vi "Record and playback example for pco.cameras with CamRam.vi"() -> ()   [LabVIEW 2012]
doc: "A short program to demonstrate the fundamentals of control and image acquision with the pco.camera series. The program records a sequence of images, with \"live\" updating, until the \"StopRecording\" button is pressed. A subset of recorded images is then read out from the camera RAM. Warning: Limit the number of images read back tfrom the camera RAM to a reasonable number. Images are stored as a three-dimensional array, which can very large. Use ctrl-H for more help on the individual controls and indicators.\n\nCopyright 2004, the Cooke Corporation."
panel:
  out "bClose":bool
  in  "Quit":bool
  in  "ImageNr":i32
  in  "Image":i32
  out "BufNr1":i16
  out "BufNr0":i16
  in  "bUseBuffer1":bool
  in  "bUseBuffer0":bool
  in  "ROIX1":u16=1 min=1
  in  "ROIY1":u16=1 min=1
  in  "ROIY0":u16=1 min=1
  in  "ROIX0":u16=1 min=1
  out "Bits/pixel":u16
  in  "Readout":bool
  in  "Record":bool
  in  "Stop":u32=10 min=1
  in  "Start":u32=1 min=1
  in  "DelayTimeBase":u16(ring)=2 items=["nanoseconds", "microseconds", "milliseconds"]
  in  "ExposureTimeBase":u16(ring)=2 items=["nanoseconds", "microseconds", "milliseconds"]
  in  "Exposure":u32=10
  in  "Delay":u32
  out "Reading":bool
  in  "StorageMode":bool
  out "ImageCount":u32
  in  "Rate":i32
  out "Image":u16[][](graph)
  in  "TriggerMode":u16(ring) items=["Auto", "Software", "External sequence start ", "External exposure control"]
  # "A short program to demonstrate the fundamentals of control and image acquision with the pco.camera series. The program records a sequence of images, with \"live\" updating, until the \"StopRecording\" button is pressed. A subset of recorded images is then read out from the camera RAM. WARNING: Limit the number of images read back tfrom the camera RAM to a reasonable number. Images are stored as a three-dimensional array, which can very large.  Use ctrl-H for more help on the individual controls and indicators."
  # "pco.labview"
  # "1) Setup camera:"
  # "FIFO"
  # "Recorder"
  # "2) Record  images:"
  # "3) Read out images:"
  # "4) Display image:"
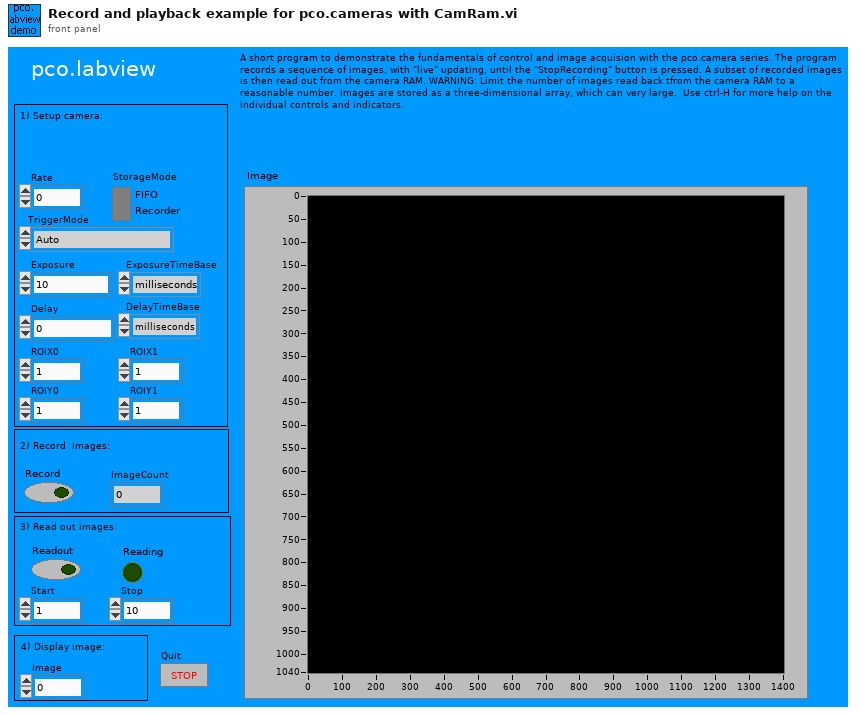
[diagram p1: front panel]
types:
  T1 = cluster{"Size":u16, "CamType":u16, "CamSubType":u16, "SerialNumber":u32, "HWVersion":u32, "FWVersion":u32, "InterfaceType":u16, "HardwareVersion":cluster{"BoardNum":u16, "HWVersions":cluster{"BoardName":string, "BatchNumber":u16, "MinorRevision":u8, "MajorRevision":u8, "Variant":u16}[]}, "FirmwareVersion":cluster{"DeviceNum":u16, "FWVersions":cluster{"DeviceName":string, "MinorRevision":u8, "MajorRevision":u8, "Variant":u16}[]}}
  T2 = cluster{"Size":u16, "SensorTypeDESC":u16, "SensorSubtypeDESC":u16, "MaxHorizontalResStdDESC":u16, "MaxVerticalResStdDESC":u16, "MaxHorizontalResExtDESC":u16, "MaxVerticalResExtDESC":u16, "DynResDESC":u16, "MaxBinHorzDESC":u16, "BinHorzStepDESC":bool, "MaxBinVertDESC":u16, "BinVertStepDESC":bool, "ROIHorzStepDESC":u16, "ROIVertStepDESC":u16, "NumADCDESC":u16, "IRDESC":bool, "MinDelayDESC":u32, "MaxDelayDESC":u32, "MinDelayStepDESC":u32, "MinExpoDESC":u32, "MaxExpoDESC":u32, "MinExpoStepDESC":u32, "MinDelayIRDESC":u32, "MaxDelayIRDESC":u32, "MinExpoIRDESC":u32, "MaxExpoIRDESC":u32, "TimeTableDESC":bool, "DoubleImageDESC":bool, "MinCoolSetDESC":i16, "MaxCoolSetDESC":i16, "MDefaultCoolSetDESC":i16, "PowerDownModeDESC":bool, "OffsetRegDESC":bool, "ColorPattern":cluster{"UpperLeftColor":u8, "UpperRightColor":u8, "LowerLeftColor":u8, "LowerRightColor":u8}, "PatternTypeDESC":bool, "PixelRates":u32[], "CoversionFactors":u16[], "Reserved":u32[], "NoiseFilterCapable":bool, "HotPixelCapable":bool, "HotPixelWithNoiseFilter":bool, "ASCIITimeCapable":bool, "Extended Description":bool, "Get Extended":bool, "Reserved Flag 1":bool, "Reserved Flag 2":bool}
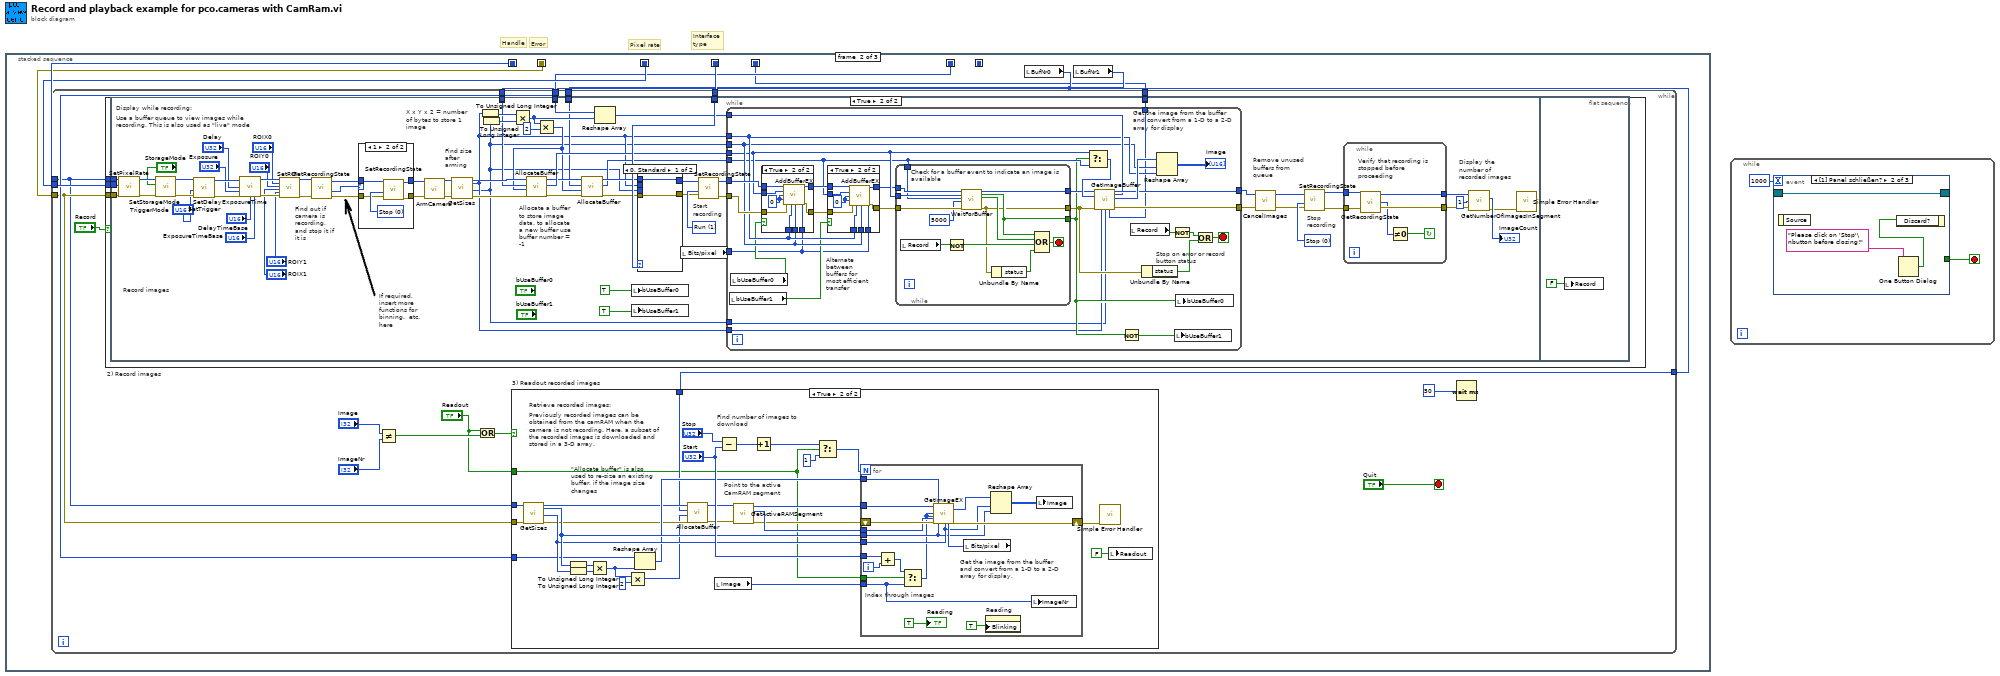
[diagram p0: block diagram]
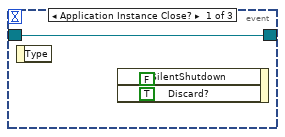
[diagram p2: hidden frame]
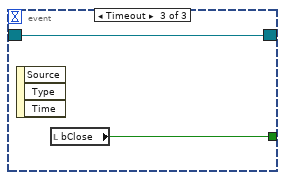
[diagram p3: hidden frame]
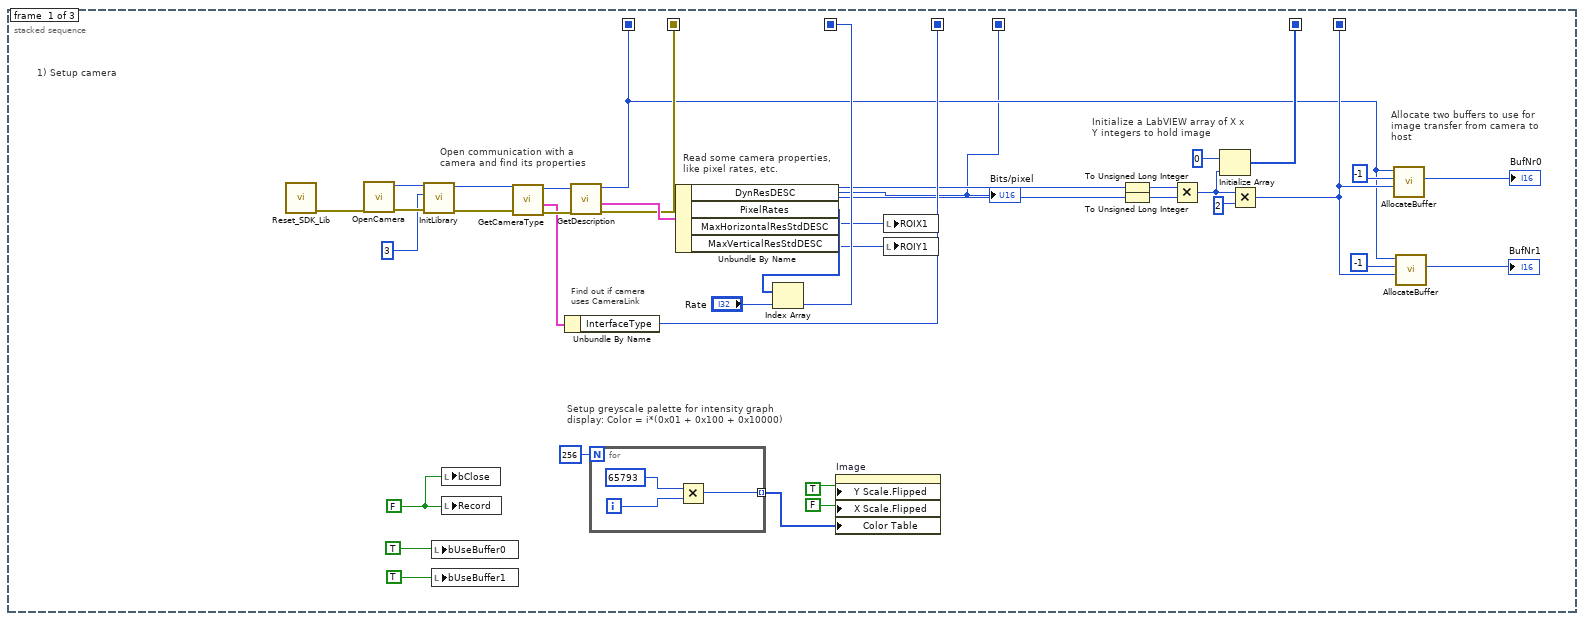
[diagram p4: hidden frame]
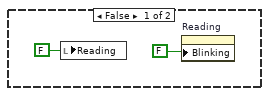
[diagram p5: hidden frame]
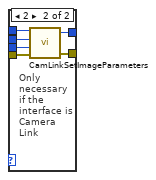
[diagram p9: hidden frame]
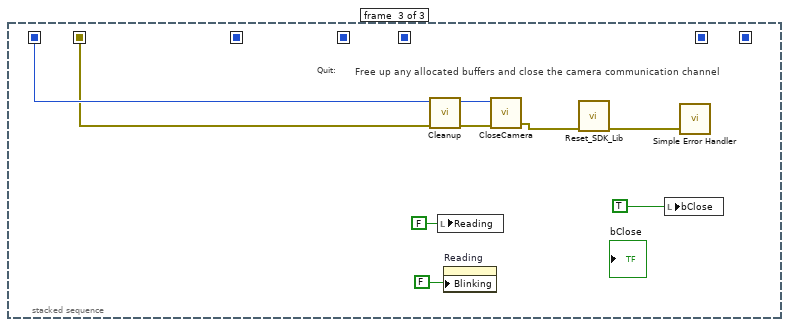
[diagram p11: hidden frame]
diagram:
  # "Interface type"
  # "Error"
  # "Handle"
  # "Pixel rate"
  n1 = stacked-sequence {
    seq-local: [w31 _ _] -> [_ w44 _]
    seq-local: [w15 _ _] -> [_ _ _]
    seq-local: [w23 _ _] -> [_ w46 _]
    seq-local: [w14 _ _] -> [_ w48 w285]
    seq-local: [w22 _ _] -> [_ w47 w284]
    seq-local: [w21 _ _] -> [_ w45 _]
    seq-local: [w1 _ _] -> [_ w41 _]
    frame #0 {
      w8 = FALSE ("stop")
      # "Read some camera properties, like pixel rates, etc."
      # "Allocate two buffers to use for image transfer from camera to host"
      # "1) Setup camera"
      # "Find out if camera uses CameraLink"
      # "Setup greyscale palette for intensity graph display: Color = i*(0x01 + 0x100 + 0x10000)"
      # "Initialize a LabVIEW array of X x Y integers to hold image"
      # "Open communication with a camera and find its properties"
      n2 = call "Reset_SDK_Lib.vi"() -> ("ErrorOut"=w4:errorcluster)  [unwired: 11 in]
      n3 = call "OpenCamera.vi"("ErrorIn"=w4) -> ("ErrorOut"=w6:errorcluster, "Handle out"=w7:u64)  [unwired: 3 in, 2 out]
      n4 = call "InitLibrary.vi"("error in (no error)"=w6, "InterfaceType"=u32 3, "ph"=w7) -> ("error out"=w2:errorcluster, "hout"=w3:u64)  [unwired: 7 in]
      n5 = local write "bUseBuffer0"(TRUE) -> ()
      n6 = local write "bUseBuffer1"(TRUE) -> ()
      n7 = local write "bClose"(w8) -> ()
      n8 = local write "Record"(w8) -> ()
      n9 = call "GetCameraType.vi"("ph"=w3, "error in (no error)"=w2) -> ("hout"=w27:u64, "CameraType"=w25:T1, "error out"=w26:errorcluster)  [unwired: 1 in, 1 out]
      n10 = Unbundle By Name(w25) -> ("InterfaceType"=w21:u16)
      n11 = call "GetDescription.vi"("ErrorIn"=w26, "ph"=w27) -> ("ErrorOut"=w22:errorcluster, "Description"=w30:T2, "hout"=w14:u64)  [unwired: 2 in, 1 out]
      n12 = for {
        N: 256 -> [_]
        tunnel: [w38] -> w34 mode=indexing
        i -> [w39]
        n13 = Multiply(x=65793, y=w39) -> (x*y=w38:i32)
      }
      n14 = Unbundle By Name(w30) -> ("DynResDESC"=w1:u16, "PixelRates"=w24:u32[], "MaxHorizontalResStdDESC"=w20:u16, "MaxVerticalResStdDESC"=w19:u16)
      "Bits/pixel" <- w1
      n15 = Index Array(array=w24, index="Rate") -> (element=w23:u32)
      n16 = property on="Image" class="IntGraph (strikt)"("Y Scale.Flipped"=TRUE, "X Scale.Flipped"=FALSE, "Color Table"=w34) -> ()  [unwired: 2 in, 2 out]
      n17 = local write "ROIX1"(w20) -> ()
      n18 = local write "ROIY1"(w19) -> ()
      n19 = To Unsigned Long Integer(number=w20) -> (unsigned 32bit integer=w17:u32)
      n20 = To Unsigned Long Integer(number=w19) -> (unsigned 32bit integer=w16:u32)
      n21 = Multiply(x=w17, y=w16) -> (x*y=w32:u32)
      n22 = Initialize Array(u16 0 ("Element Data"), w32) -> (w31:u16[])
      n23 = Multiply(x=w32, y=u32 2) -> (x*y=w15:u32)
      n24 = call "AllocateBuffer.vi"("Size"=w15, "BufNr"=i16 -1, "ph"=w14) -> ("BufNrOut"=→"BufNr0":i16)  [unwired: 3 in, 5 out]
      n25 = call "AllocateBuffer.vi"("Size"=w15, "BufNr"=-1, "ph"=w14) -> ("BufNrOut"=→"BufNr1":i16)  [unwired: 3 in, 5 out]
    }
    frame #1 {
      n26 = local read "BufNr0"() -> (w43:i16)
      n27 = local read "BufNr1"() -> (w42:i16)
      n28 = while {
        tunnel: w43 -> [w58]
        tunnel: w43 -> [w59]
        tunnel: w44 -> [w61]
        tunnel: w45 -> [w62]
        tunnel: w46 -> [w63]
        tunnel: w47 -> [w60]
        tunnel: w48 -> [w56]
        tunnel: w42 -> [w57]
        tunnel: w41 -> [w49]
        stop <- "Quit" stop-if-true
        n29 = case "2) Record images" shown="True" "Record" {
          tunnel: w56 -> [_ w122]
          tunnel: w60 -> [_ w121]
          tunnel: w63 -> [_ w120]
          tunnel: w62 -> [_ w119]
          tunnel: w61 -> [_ w118]
          tunnel: w59 -> [_ w117]
          tunnel: w57 -> [_ w116]
          tunnel: w49 -> [_ w115]
          frame False {
          }
          frame True {
            n30 = flat-sequence {
              tunnel: w122 -> [w166]
              tunnel: w121 -> [w165]
              tunnel: w120 -> [w163]
              tunnel: w119 -> [w162]
              tunnel: w118 -> [w160]
              tunnel: w117 -> [w145]
              tunnel: w116 -> [w139]
              tunnel: w115 -> [w123]
              frame #0 {
                w190 = u16 1 items=["Stop", "Run"] ("RecordingState")
                w193 = u16 0 items=["Stop", "Run"] ("RecordingState")
                # "Remove unused buffers from queue"
                # "Display the number of recorded images"
                # "Record images"
                # "Start recording"
                # "Allocate a buffer to store image data. to allocate a new buffer use buffer number = -1"
                # "Find size after arming"
                # "Find out if camera is recording, and stop it if it is"
                # "If required, insert more functions for binning.  etc. here"
                # "X x Y x 2 = number of bytes to store 1 image"
                # "Stop recording"
                # "Use a buffer queue to view images while recording. This is also used as \"live\" mode"
                # "Display while recording:"
                n31 = call "SetPixelRate.vi"("error in (no error)"=w165, "PixelRate"=w163, "ph"=w166) -> ("error out"=w188:errorcluster, "hout"=w189:u64)  [unwired: 2 in, 1 out]
                n32 = call "SetStorageMode.vi"("error in (no error)"=w188, "StorageMode"="StorageMode", "ph"=w189) -> ("error out"=w180:errorcluster, "hout"=w181:u64)  [unwired: 2 in, 1 out]
                n33 = call "SetTrigger.vi"("error in (no error)"=w180, "TriggerMode"="TriggerMode", "ph"=w181) -> ("error out"=w173:errorcluster, "hout"=w174:u64)  [unwired: 2 in, 1 out]
                n34 = call "SetDelayExposureTime.vi"("ph"=w174, "Delay"="Delay", "Exposure"="Exposure", "error in (no error)"=w173, "DelayTimeBase"="DelayTimeBase", "ExposureTimeBase"="ExposureTimeBase") -> ("hout"=w153:u64, "error out"=w151:errorcluster)  [unwired: 7 in, 1 out]
                n35 = call "SetROI.vi"("ph"=w153, "ROIX0"="ROIX0", "ROIY0"="ROIY0", "ROIX1"="ROIX1", "ROIY1"="ROIY1", "error in (no error)"=w151) -> ("hout"=w152:u64, "error out"=w150:errorcluster)  [unwired: 12 in]
                n36 = call "GetRecordingState.vi"("ErrorIn"=w150, "ph"=w152) -> ("ErrorOut"=w184:errorcluster, "RecordingState"=w186:u16, "hout"=w185:u64)  [unwired: 2 in, 1 out]
                n37 = case shown="1" w186 {
                  tunnel: w185 -> [w274 w278]
                  tunnel: w184 -> [w273 w277]
                  tunnel: [w274 w276] -> w183
                  tunnel: [w273 w275] -> w182
                  frame 0, Default {
                  }
                  frame 1 {
                    w279 = u16 0 items=["Stop", "Run"] ("RecordingState")
                    n38 = call "SetRecordingState.vi"("ErrorIn"=w277, "RecordingState"=w279, "ph"=w278) -> ("ErrorOut"=w275:errorcluster, "hout"=w276:u64)  [unwired: 2 in, 1 out]
                  }
                }
                n39 = call "ArmCamera.vi"("error in (no error)"=w182, "ph"=w183) -> ("error out"=w178:errorcluster, "hout"=w179:u64)  [unwired: 1 in, 1 out]
                n40 = call "GetSizes.vi"("ph"=w179, "ErrorIn"=w178) -> ("hout"=w175:u64, "XResAct"=w125:u16, "YResAct"=w124:u16, "ErrorOut"=w177:errorcluster)  [unwired: 11 in, 3 out]
                n41 = To Unsigned Long Integer(number=w125) -> (unsigned 32bit integer=w154:u32)
                n42 = To Unsigned Long Integer(number=w124) -> (unsigned 32bit integer=w155:u32)
                n43 = Multiply(x=w154, y=w155) -> (x*y=w156:u32)
                n44 = Multiply(x=w156, y=u32 2) -> (x*y=w140:u32)
                n45 = call "AllocateBuffer.vi"("error in (no error)"=w177, "Size"=w140, "BufNr"=w145, "ph"=w175) -> ("error out"=w144:errorcluster, "BufNrOut"=w157:i16, "hout"=w142:u64)  [unwired: 2 in, 3 out]
                n46 = call "AllocateBuffer.vi"("error in (no error)"=w144, "Size"=w140, "BufNr"=w139, "ph"=w142) -> ("error out"=w143:errorcluster, "BufNrOut"=w138:i16, "hout"=w141:u64)  [unwired: 2 in, 3 out]
                n47 = Reshape Array(w160, w156) -> (w159:u16[])
                n48 = local write "bUseBuffer0"(TRUE) -> ()
                n49 = local write "bUseBuffer1"(TRUE) -> ()
                n50 = case shown="0, Standard" w162 {
                  tunnel: w143 -> [w265 w272]
                  tunnel: [w265 w271] -> w168
                  tunnel: w141 -> [w266 w270]
                  tunnel: [w266 w269] -> w167
                  tunnel: w124 -> [_ w268]
                  tunnel: w125 -> [_ w267]
                  frame 0, Default {
                  }
                  frame 2 {
                    # "Only necessary if the interface is Camera Link"
                    n51 = call "CamLinkSetImageParameters.vi"("error in (no error)"=w272, "YRes"=w268, "XRes"=w267, "ph"=w270) -> ("error out"=w271:errorcluster, "hout"=w269:u64)  [unwired: 1 out]
                  }
                }
                n52 = local read "Bits/pixel"() -> (w131:u16)
                n53 = call "SetRecordingState.vi"("ErrorIn"=w168, "RecordingState"=w190, "ph"=w167) -> ("ErrorOut"=w164:errorcluster, "hout"=w161:u64)  [unwired: 2 in, 1 out]
                n54 = while {
                  tunnel: w157 -> [w206]
                  tunnel: w159 -> [w219]
                  tunnel: w161 -> [w218]
                  tunnel: w124 -> [w213]
                  tunnel: w125 -> [w214]
                  tunnel: w164 -> [w216]
                  tunnel: [w221] -> w130
                  tunnel: [w222] -> w129
                  tunnel: w138 -> [w205]
                  tunnel: w131 -> [w209]
                  tunnel: w125 -> [w196]
                  tunnel: w124 -> [w195]
                  tunnel: w123 -> [w194]
                  stop <- w197 stop-if-true
                  # "Alternate between buffers for most efficient transfer"
                  # "Stop on error or record button status"
                  # "Get the image from the buffer and convert from a 1-D to a 2-D array for display"
                  n55 = local read "bUseBuffer1"() -> (w211:bool)
                  n56 = local read "bUseBuffer0"() -> (w212:bool)
                  n57 = case shown="True" w212 {
                    tunnel: [w225 w234] -> w215
                    tunnel: [w224 w233] -> w217
                    tunnel: w206 -> [_ w232]
                    tunnel: w218 -> [w224 w231]
                    tunnel: w209 -> [_ w229]
                    tunnel: w214 -> [_ w228]
                    tunnel: w213 -> [_ w227]
                    tunnel: w216 -> [w225 w226]
                    frame False {
                    }
                    frame True {
                      w230 = 0
                      n58 = call "AddBufferEX.vi"("ph"=w231, "BuffNr"=w232, "1stImage"=w230, "LastImage"=w230, "error in (no error)"=w226, "XRes"=w228, "YRes"=w227, "BitPerPixel"=w229) -> ("hout"=w233:u64, "error out"=w234:errorcluster)  [unwired: 5 in, 1 out]
                    }
                  }
                  n59 = case shown="True" w211 {
                    tunnel: [w235 w245] -> w203
                    tunnel: [w236 w244] -> w204
                    tunnel: w205 -> [_ w243]
                    tunnel: w217 -> [w236 w242]
                    tunnel: w209 -> [_ w240]
                    tunnel: w214 -> [_ w239]
                    tunnel: w213 -> [_ w238]
                    tunnel: w215 -> [w235 w237]
                    frame False {
                    }
                    frame True {
                      w241 = 0
                      n60 = call "AddBufferEX.vi"("ph"=w242, "BuffNr"=w243, "1stImage"=w241, "LastImage"=w241, "error in (no error)"=w237, "XRes"=w239, "YRes"=w238, "BitPerPixel"=w240) -> ("hout"=w244:u64, "error out"=w245:errorcluster)  [unwired: 5 in, 1 out]
                    }
                  }
                  n61 = while {
                    tunnel: w206 -> [w253]
                    tunnel: w205 -> [w252]
                    tunnel: w204 -> [w255]
                    tunnel: w203 -> [w254]
                    tunnel: [w251] -> w202
                    tunnel: [w247] -> w200
                    tunnel: [w250] -> w201
                    stop <- w256 stop-if-true
                    # "Check for a buffer event to indicate an image is available"
                    n62 = local read "Record"() -> (w258:bool)
                    n63 = Not(x=w258) -> (.not. x?=w257:bool)
                    n64 = call "WaitForBuffer.vi"("ph"=w255, "sBufNr"=w253, "sBufNr 2"=w252, "timeout"=5000, "error in (no error)"=w254) -> ("hout"=w251:u64, "Buffer_Ready"=w250:bool, "Buffer_Ready 2"=w249:bool, "error out"=w247:errorcluster)  [unwired: 10 in, 1 out]
                    n65 = Unbundle By Name(w247) -> ("status"=w246:bool)
                    n66 = Compound Arithmetic op=OR(w250, w249, w257, w246) -> (w256:bool)
                  }
                  n67 = Select(t=w206, s=w201, f=w205) -> (s? t:f=w210:i16)
                  n68 = call "GetImageBuffer.vi"("ph"=w202, "BuffIn"=w219, "BuffNr"=w210, "error in (no error)"=w200, "xRes"=w196, "yRes"=w195, "Bitresolution"=w194) -> ("hout"=w221:u64, "BuffOut"=w223:u16[], "error out"=w222:errorcluster)  [unwired: 5 in, 1 out]
                  n69 = Not(x=w201) -> (.not. x?=w208:bool)
                  n70 = local read "Record"() -> (w220:bool)
                  n71 = Unbundle By Name(w200) -> ("status"=w198:bool)
                  n72 = Reshape Array(w223, w213, w214) -> (→"Image":u16[][])
                  n73 = Not(x=w220) -> (.not. x?=w199:bool)
                  n74 = local write "bUseBuffer1"(w208) -> ()
                  n75 = local write "bUseBuffer0"(w201) -> ()
                  n76 = Or(x=w199, y=w198) -> (x .or. y?=w197:bool)
                }
                n77 = call "CancelImages.vi"("error in (no error)"=w129, "ph"=w130) -> ("error out"=w135:errorcluster, "hout"=w134:u64)  [unwired: 1 in, 1 out]
                n78 = call "SetRecordingState.vi"("ErrorIn"=w135, "RecordingState"=w193, "ph"=w134) -> ("ErrorOut"=w191:errorcluster, "hout"=w192:u64)  [unwired: 2 in, 1 out]
                n79 = while {
                  tunnel: [w262] -> w128
                  tunnel: w191 -> [w263]
                  tunnel: w192 -> [w264]
                  tunnel: [w259] -> w127
                  stop <- w260 continue-if-true
                  # "Verify that recording is stopped before proceeding"
                  n80 = call "GetRecordingState.vi"("ErrorIn"=w263, "ph"=w264) -> ("ErrorOut"=w262:errorcluster, "RecordingState"=w261:u16, "hout"=w259:u64)  [unwired: 2 in, 1 out]
                  n81 = Not Equal To 0?(x=w261) -> (x != 0?=w260:bool)
                }
                n82 = call "GetNumberOfImagesInSegment.vi"("ph"=w127, "Segment"=u16 1, "error in (no error)"=w128) -> ("ValidImageCnt"=→"ImageCount":u32, "error out"=w126:errorcluster)  [unwired: 3 out]
                n83 = call <vilib>:"Simple Error Handler.vi"("error in (no error)"=w126) -> ()  [unwired: 4 in, 5 out]
              }
              frame #1 {
                n84 = local write "Record"(FALSE ("Record")) -> ()
              }
            }
          }
        }
        n85 = Not Equal?(x="Image", y="ImageNr") -> (x != y?=w53:bool)
        n86 = Or(x="Readout", y=w53) -> (x .or. y?=w52:bool)
        n87 = case "3) Readout recorded images" shown="True" w52 {
          tunnel: w61 -> [_ w89]
          tunnel: w56 -> [_ w81]
          tunnel: w60 -> [_ w80]
          tunnel: w58 -> [_ w74]
          tunnel: "Readout" -> [_ w68]
          frame False {
            n88 = local write "Reading"(FALSE ("Reading")) -> ()
            n89 = property on="Reading" class="Bool. (strikt)"("Blinking"=FALSE) -> ()  [unwired: 2 in, 2 out]
          }
          frame True {
            # "Point to the active CamRAM segment"
            # "\"Allocate buffer\" is also used to re-size an existing buffer, if the image size changes"
            # "Find number of images to download"
            # "Previously recorded images can be obtained from the camRAM when the camera is not recording. Here, a subset of the recorded images is downloaded and stored in a 3-D array."
            # "Retrieve recorded images:"
            n90 = call "GetSizes.vi"("ph"=w81, "ErrorIn"=w80) -> ("hout"=w87:u64, "XResAct"=w91:u16, "YResAct"=w90:u16, "ErrorOut"=w85:errorcluster)  [unwired: 11 in, 3 out]
            n91 = To Unsigned Long Integer(number=w91) -> (unsigned 32bit integer=w77:u32)
            n92 = To Unsigned Long Integer(number=w90) -> (unsigned 32bit integer=w78:u32)
            n93 = Multiply(x=w77, y=w78) -> (x*y=w79:u32)
            n94 = Multiply(x=w79, y=u32 2) -> (x*y=w76:u32)
            n95 = Reshape Array(w89, w79) -> (w88:u16[])
            n96 = call "AllocateBuffer.vi"("error in (no error)"=w85, "Size"=w76, "BufNr"=w74, "ph"=w87) -> ("error out"=w84:errorcluster, "hout"=w86:u64)  [unwired: 2 in, 4 out]
            n97 = local read "Image"() -> (w72:i32)
            n98 = Subtract(x="Stop", y="Start") -> (x-y=w95:u32)
            n99 = call "GetActiveRAMSegment.vi"("error in (no error)"=w84, "ph"=w86) -> ("error out"=w82:errorcluster, "ActSeg"=w92:u16, "hout"=w83:u64)  [unwired: 2 in, 1 out]
            n100 = Increment(x=w95) -> (x+1=w71:u32)
            n101 = Select(t=w71, s=w68, f=1) -> (s? t:f=w70:u32)
            n102 = for {
              N: w70 -> [_]
              tunnel: w83 -> [w114]
              shift-right: [w111] -> w73
              shift-left: w82 -> [w110]
              tunnel: "Start" -> [w107]
              tunnel: w92 -> [w105]
              tunnel: w91 -> [w101]
              tunnel: w90 -> [w102]
              tunnel: w88 -> [w103]
              tunnel: w72 -> [w97]
              tunnel: w68 -> [w99]
              i -> [w106]
              # "Get the image from the buffer and convert from a 1-D to a 2-D array for display."
              # "Index through images"
              n103 = Add(x=w107, y=w106) -> (x+y=w98:u32)
              n104 = Select(t=w98, s=w99, f=w97) -> (s? t:f=w100:u32)
              n105 = local read "Bits/pixel"() -> (w104:u16)
              n106 = call "GetImageEX.vi"("ph"=w114, "1stImage"=w100, "lastImage"=w100, "segment"=w105, "error in (no error)"=w110, "BuffIn"=w103, "xRes"=w101, "yRes"=w102, "BitPerPixel"=w104) -> ("BuffOut"=w113:u16[], "error out"=w111:errorcluster)  [unwired: 7 in, 2 out]
              n107 = property on="Reading" class="Bool. (strikt)"("Blinking"=TRUE) -> ()  [unwired: 2 in, 2 out]
              n108 = Reshape Array(w113, w102, w101) -> (w112:u16[][])
              n109 = local write "ImageNr"(w97) -> ()
              n110 = local write "Image"(w112) -> ()
              "Reading" <- TRUE ("Reading")
            }
            n111 = call <vilib>:"Simple Error Handler.vi"("error in (no error)"=w73) -> ()  [unwired: 4 in, 5 out]
            n112 = local write "Readout"(FALSE ("Readout")) -> ()
          }
        }
        n113 = Wait (ms)(milliseconds to wait=u32 50) -> ()  [unwired: 1 out]
      }
    }
    frame #2 {
      # "Free up any allocated buffers and close the camera communication channel"
      # "Quit:"
      n114 = call "Cleanup.vi"("error in (no error)"=w284, "ph"=w285) -> ("error out"=w283:errorcluster, "hout"=w282:u64)  [unwired: 8 in]
      n115 = local write "Reading"(FALSE ("Reading")) -> ()
      n116 = property on="Reading" class="Bool. (strikt)"("Blinking"=FALSE) -> ()  [unwired: 2 in, 2 out]
      n117 = call "CloseCamera.vi"("ErrorIn"=w283, "Handle in"=w282) -> ("ErrorOut"=w281:errorcluster)  [unwired: 1 in, 2 out]
      n118 = call "Reset_SDK_Lib.vi"("ErrorIn"=w281) -> ("ErrorOut"=w286:errorcluster)  [unwired: 10 in]
      n119 = local write "bClose"(TRUE) -> ()
      n120 = call <vilib>:"Simple Error Handler.vi"("error in (no error)"=w286) -> ()  [unwired: 4 in, 5 out]
    }
  }
  n121 = while {
    stop <- w290 stop-if-true
    n122 = event shown="[1] Panel schließen?" {
      selector: _ -> [w292 w297 w299]
      dyn-events: [w292 w297 w299] -> _
      timeout: 1000 -> [_ _ _]
      tunnel: [_ _ w298] -> w290
      event Application Instance Close? {
        n123 = event-data() -> ()  [unwired: 1 in, 1 out]
        n124 = event-data("SilentShutdown"=FALSE, "Discard?"=TRUE) -> ()  [unwired: 1 in, 1 out]
      }
      event Panel Close? {
        n125 = event-data() -> ()  [unwired: 1 in, 1 out]
        n126 = One Button Dialog(message="Please click on 'Stop'\nbutton before closing!") -> (true=w295:bool)  [unwired: 1 in]
        n127 = event-data("Discard?"=w295) -> ()  [unwired: 1 in, 1 out]
      }
      event Timeout {
        n128 = event-data() -> ()  [unwired: 1 in, 3 out]
        n129 = local read "bClose"() -> (w298:bool)
      }
    }
  }
